vi "Logic-CheckToDeleteData.vi"(8 "error in (no error)":errorcluster, 11 "TableLogger Config":T1) -> (0 "error out":errorcluster, 3 "Deleted?T":bool)   [LabVIEW 2014, in "TableLogger_SQLite_Actor.lvlib" / "TableLogger_SQLite_Actor.lvclass"]
uses:
  TableLogger_SQLite_Actor.lvclass
  TableLogger_Actor/TableLoggerConfig.ctl
  TableLogger_Actor/TableLoggerTypes.ctl
  TableLogger_Actor/TableLoggerBackupConfig.ctl
  TableLogger_Actor/TableLogger_Actor.lvlib
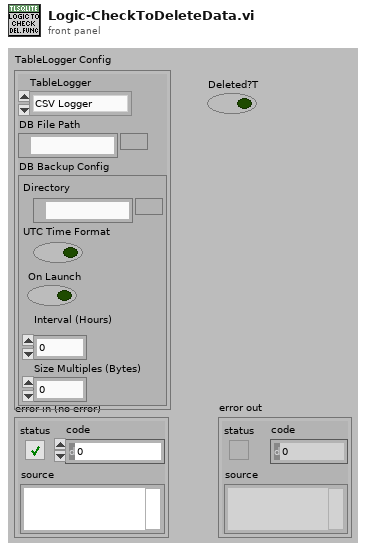
[diagram p1: front panel]
types:
  T1 = typedef "TableLogger_Actor.lvlib/TableLoggerConfig.ctl" = cluster{"TableLogger":T2, "DB File Path":path, "DB Backup Config":T3}
  T2 = typedef "TableLogger_Actor.lvlib/TableLoggerTypes.ctl" = enum16{"CSV Logger", "SQLite Logger"}
  T3 = typedef "TableLogger_Actor.lvlib/TableLoggerBackupConfig.ctl" = cluster{"Directory":path, "UTC Time Format":bool, "On Launch":bool, "Interval (Hours)":dbl, "Size Multiples (Bytes)":i32}
  T4 = cluster{"Numeric Data":i32, "Float Data":dbl, "String Data":string, "Enum Data":enum16{"Enum Item 1", "Enum Item 2"}, "Array Data":i32[], "Array Data 2":i32[], "Numeric Data 2":i32, "Array Data 3":i32[]}[]
  T5 = cluster{"Numeric Data":i32, "Float Data":dbl, "String Data":string, "Enum Data":enum16{"Enum Item 1", "Enum Item 2"}, "Array Data":i32[]}
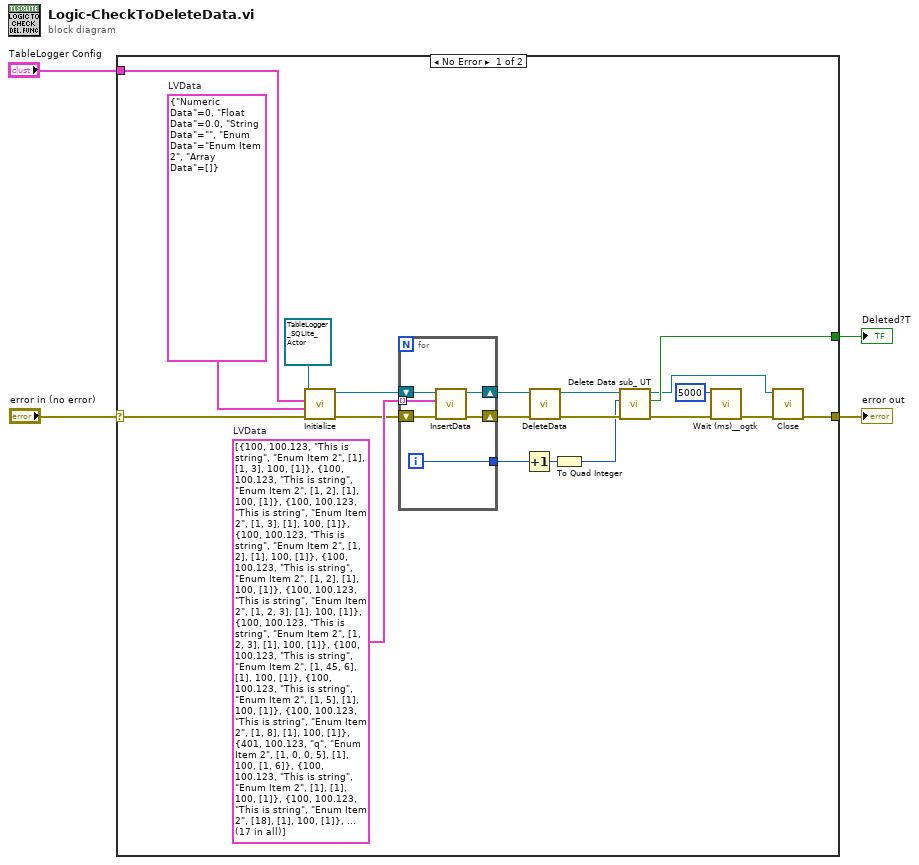
[diagram p0: block diagram]
diagram:
  n1 = case shown="No Error" "error in (no error)" {
    selector: "error in (no error)" -> [w19 w31]
    tunnel: [w24 _] -> w4
    tunnel: [w9 w31] -> w2
    tunnel: "TableLogger Config" -> [w8 _]
    frame No Error {
      w21 = T4 [{"Numeric Data"=100, "Float Data"=100.123, "String Data"="This is string", "Enum Data"=enum."Enum Item 2", "Array Data"=[1], "Array Data 2"=[1, 3], "Numeric Data 2"=100, "Array Data 3"=[1]}, {"Numeric Data"=100, "Float Data"=100.123, "String Data"="This is string", "Enum Data"=enum."Enum Item 2", "Array Data"=[1, 2], "Array Data 2"=[1], "Numeric Data 2"=100, "Array Data 3"=[1]}, {"Numeric Data"=100, "Float Data"=100.123, "String Data"="This is string", "Enum Data"=enum."Enum Item 2", "Array Data"=[1, 3], "Array Data 2"=[1], "Numeric Data 2"=100, "Array Data 3"=[1]}, {"Numeric Data"=100, "Float Data"=100.123, "String Data"="This is string", "Enum Data"=enum."Enum Item 2", "Array Data"=[1, 2], "Array Data 2"=[1], "Numeric Data 2"=100, "Array Data 3"=[1]}, {"Numeric Data"=100, "Float Data"=100.123, "String Data"="This is string", "Enum Data"=enum."Enum Item 2", "Array Data"=[1, 2], "Array Data 2"=[1], "Numeric Data 2"=100, "Array Data 3"=[1]}, {"Numeric Data"=100, "Float Data"=100.123, "String Data"="This is string", "Enum Data"=enum."Enum Item 2", "Array Data"=[1, 2, 3], "Array Data 2"=[1], "Numeric Data 2"=100, "Array Data 3"=[1]}, {"Numeric Data"=100, "Float Data"=100.123, "String Data"="This is string", "Enum Data"=enum."Enum Item 2", "Array Data"=[1, 2, 3], "Array Data 2"=[1], "Numeric Data 2"=100, "Array Data 3"=[1]}, {"Numeric Data"=100, "Float Data"=100.123, "String Data"="This is string", "Enum Data"=enum."Enum Item 2", "Array Data"=[1, 45, 6], "Array Data 2"=[1], "Numeric Data 2"=100, "Array Data 3"=[1]}, {"Numeric Data"=100, "Float Data"=100.123, "String Data"="This is string", "Enum Data"=enum."Enum Item 2", "Array Data"=[1, 5], "Array Data 2"=[1], "Numeric Data 2"=100, "Array Data 3"=[1]}, {"Numeric Data"=100, "Float Data"=100.123, "String Data"="This is string", "Enum Data"=enum."Enum Item 2", "Array Data"=[1, 8], "Array Data 2"=[1], "Numeric Data 2"=100, "Array Data 3"=[1]}, {"Numeric Data"=401, "Float Data"=100.123, "String Data"="q", "Enum Data"=enum."Enum Item 2", "Array Data"=[1, 0, 0, 5], "Array Data 2"=[1], "Numeric Data 2"=100, "Array Data 3"=[1, 6]}, {"Numeric Data"=100, "Float Data"=100.123, "String Data"="This is string", "Enum Data"=enum."Enum Item 2", "Array Data"=[1], "Array Data 2"=[1], "Numeric Data 2"=100, "Array Data 3"=[1]}, {"Numeric Data"=100, "Float Data"=100.123, "String Data"="This is string", "Enum Data"=enum."Enum Item 2", "Array Data"=[18], "Array Data 2"=[1], "Numeric Data 2"=100, "Array Data 3"=[1]}, {"Numeric Data"=100, "Float Data"=100.123, "String Data"="This is string", "Enum Data"=enum."Enum Item 2", "Array Data"=[1, 0, 0, 0, 98], "Array Data 2"=[1], "Numeric Data 2"=100, "Array Data 3"=[1]}, {"Numeric Data"=100, "Float Data"=100.123, "String Data"="This is string", "Enum Data"=enum."Enum Item 2", "Array Data"=[1, 2], "Array Data 2"=[1, 2], "Numeric Data 2"=100, "Array Data 3"=[1]}, {"Numeric Data"=100, "Float Data"=100.123, "String Data"="This is string", "Enum Data"=enum."Enum Item 2", "Array Data"=[1, 2, 2], "Array Data 2"=[1], "Numeric Data 2"=100, "Array Data 3"=[1]}, {"Numeric Data"=100, "Float Data"=100.123, "String Data"="This is string", "Enum Data"=enum."Enum Item 2", "Array Data"=[1], "Array Data 2"=[1, 1], "Numeric Data 2"=100, "Array Data 3"=[1]}]  # LVData
      w12 = T5 {"Numeric Data"=0, "Float Data"=0.0, "String Data"="", "Enum Data"=enum."Enum Item 2", "Array Data"=[]}  # LVData
      n2 = call-dynamic "Initialize.vi"("error in (no error)"=w19, "Data Cluster (for Table Headers)"=w12, "TableLogger Config"=w8, "object in"=refnum<class "TableLogger_SQLite_Actor.lvclass"> refnum) -> ("error out"=w17:errorcluster, "object out"=w15:refnum<class "TableLogger_SQLite_Actor.lvclass">)  [unwired: 6 in]
      n3 = for {
        shift-right: [w29] -> w18
        shift-left: w17 -> [w30]
        shift-right: [w27] -> w16
        shift-left: w15 -> [w28]
        tunnel: w21 -> [w26] mode=indexing
        tunnel: [w25] -> w7
        i -> [w25]
        n4 = call-dynamic "InsertData.vi"("error in (no error)"=w30, "Data Cluster"=w26, "object in"=w28) -> ("error out"=w29:errorcluster, "object out"=w27:refnum<class "TableLogger_SQLite_Actor.lvclass">)  [unwired: 7 in]
      }
      n5 = Increment(x=w7) -> (x+1=w6:i32)
      n6 = call-dynamic "DeleteData.vi"("error in (no error)"=w18, "object in"=w16) -> ("error out"=w20:errorcluster, "object out"=w22:refnum<class "TableLogger_SQLite_Actor.lvclass">)  [unwired: 7 in, 1 out]
      n7 = To Quad Integer(1:w6) -> (0:w5:i64)
      n8 = call "Delete Data sub_ UT.vi"("error in (no error)"=w20, "No. of Rows"=w5, "TableLogger_SQLite_Actor in"=w22) -> ("error out"=w10:errorcluster, "Deleted?T"=w24:bool, "TableLogger_SQLite_Actor out"=w23:refnum<class "TableLogger_SQLite_Actor.lvclass">)  [unwired: 6 in]
      n9 = call <userlib>:"Wait (ms)__ogtk.vi"("error in (no error)"=w10, "milliseconds to wait"=u32 5000) -> ("error out"=w13:errorcluster)  [unwired: 8 in, 1 out]
      n10 = call-dynamic "Close.vi"("error in (no error)"=w13, "object in"=w23) -> ("error out"=w9:errorcluster)  [unwired: 8 in, 1 out]
    }
    frame Error {
    }
  }
  "Deleted?T" <- w4
  "error out" <- w2
